vi "perfer given heading.vi"(9 "desired heading":i8, 10 "min obstacle dist":u16, 11 "driveable path lengths":u16[](array[numeric])=[0, 0, 0, 0, 0, 0, 0, 0, 0, 0, 0, 0, 0, 0, 0, 0]) -> (0 "driveable paths?":bool, 3 "wheel angle":i8)   [LabVIEW 2009]
panel:
  out "coerced x":i8
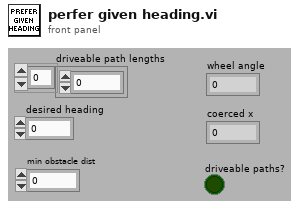
[diagram p1: front panel]
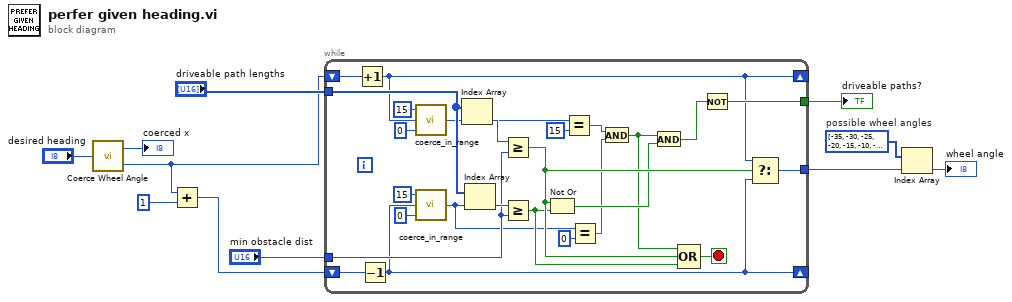
[diagram p0: block diagram]
diagram:
  w8 = i8[] [-35, -30, -25, -20, -15, -10, -5, -1, 1, 5, 10, 15, 20, 25, 30, 35]  # possible wheel angles
  n1 = call "Coerce Wheel Angle.vi"("Angle In"="desired heading") -> ("Wheel Angle"=→"coerced x":i8, "Path Index"=w1:i32)
  n2 = Add(x=w1, y=i8 1) -> (x+y=w2:i32)
  n3 = while {
    tunnel: "driveable path lengths" -> [w37]
    tunnel: "min obstacle dist" -> [w34]
    tunnel: [w31] -> w10
    shift-right: [w24] -> _
    shift-left: w1 -> [w27]
    shift-right: [w19] -> _
    shift-left: w2 -> [w26]
    tunnel: [w25] -> w9
    stop <- w32 stop-if-true
    n4 = Increment(x=w27) -> (x+1=w24:i32)
    n5 = Decrement(x=w26) -> (x-1=w19:i32)
    n6 = call "coerce_in_range.vi"("min"=i8 0, "x"=w24, "max"=i8 15) -> ("coerced x"=w18:i8)  [unwired: 2 in]
    n7 = call "coerce_in_range.vi"("min"=i8 0, "x"=w19, "max"=i8 15) -> ("coerced x"=w14:i8)  [unwired: 2 in]
    n8 = Index Array(array=w37, index=w18) -> (element=w35:u16)
    n9 = Index Array(array=w37, index=w14) -> (element=w36:u16)
    n10 = Greater Or Equal?(x=w35, y=w34) -> (x >= y?=w30:bool)
    n11 = Greater Or Equal?(x=w36, y=w34) -> (x >= y?=w29:bool)
    n12 = Not Or(1:w29, 2:w30) -> (0:w28:bool)
    n13 = Equal?(x=w18, y=15) -> (x = y?=w17:bool)
    n14 = Equal?(x=w14, y=0) -> (x = y?=w13:bool)
    n15 = And(x=w17, y=w13) -> (x .and. y?=w12:bool)
    n16 = And(x=w12, y=w28) -> (x .and. y?=w16:bool)
    n17 = Compound Arithmetic op=OR(w12, w30, w29) -> (w32:bool)
    n18 = Not(x=w16) -> (.not. x?=w31:bool)
    n19 = Select(t=w24, s=w30, f=w19) -> (s? t:f=w25:i32)
  }
  "driveable paths?" <- w10
  n20 = Index Array(array=w8, index=w9) -> (element=→"wheel angle":i8)
